vi "Engine In - Sensor - Rail Pressure.vi"(10 "Loop Freq (Hz)":sgl, 11 "Rail Pressure [V]":sgl) -> (3 "Rail Pressure [bar]":sgl)   [LabVIEW 2015, in "ECS-RT.lvlib"]
uses:
  ECS-RT.lvlib
  <vilib>/ptbypt/NI_PtbyPt.lvlib
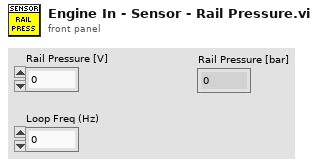
[diagram p1: front panel]
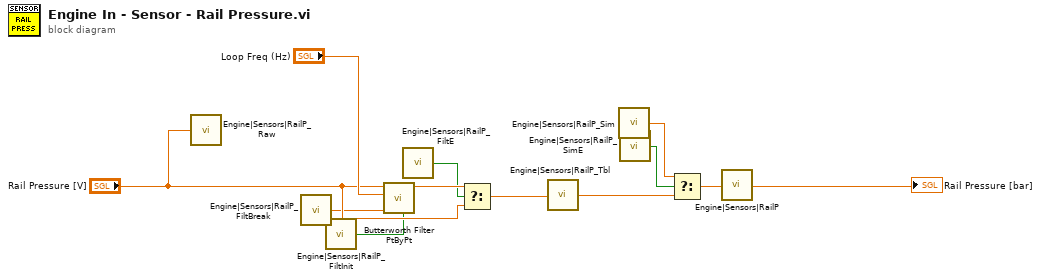
[diagram p0: block diagram]
diagram:
  n1 = call "Engine|Sensors|RailP_Raw"("Value"="Rail Pressure [V]") -> ()
  n2 = call "Engine|Sensors|RailP_FiltBreak"() -> ("Value"=w5:sgl)
  n3 = call "Engine|Sensors|RailP_FiltInit"() -> ("Value"=w8:bool)
  n4 = call <vilib>:"Butterworth Filter PtByPt.vi"("initialize"=w8, "low cutoff freq: fl"=w5, "sampling freq: fs"="Loop Freq (Hz)", "x"="Rail Pressure [V]") -> ("Filtered x"=w7:dbl)  [unwired: 5 in, 1 out]
  n5 = call "Engine|Sensors|RailP_FiltE"() -> ("Value"=w4:bool)
  n6 = Select(t=w7, s=w4, f="Rail Pressure [V]") -> (s? t:f=w6:dbl)
  n7 = call "Engine|Sensors|RailP_Tbl"("X Index"=w6) -> ("Y"=w3:sgl)
  n8 = call "Engine|Sensors|RailP_Sim"() -> ("Value"=w9:sgl)
  n9 = call "Engine|Sensors|RailP_SimE"() -> ("Value"=w2:bool)
  n10 = Select(t=w9, s=w2, f=w3) -> (s? t:f=w1:sgl)
  "Rail Pressure [bar]" <- w1
  n11 = call "Engine|Sensors|RailP"("Value"=w1) -> ()
